vi "Project Data Initial before auto.vi"(10 "VISA resource name":refnum<visa-resource-name>="COM1", 11 "configuration file path":path=path "C:/Users/MyUser/Desktop/S2_Project.txt") -> (0 "error out":errorcluster, 1 "Step Content":string[][](table), 2 "Retry":i32, 3 "process cluster":cluster{string[], i32[]})   [LabVIEW 2019]
uses:
  <vilib>/Utility/config.llb/Read Key (String).vi
  Global/Process Global.vi
  <vilib>/Utility/config.llb/NI_LVConfig.lvlib
  Ctrl/StationCmdSelect.ctl
  FlowCtrl Class/LineScan/LineScan.lvclass
  Ctrl/MeasureDisplayTab.ctl
  LLB/Commonly VI/Main Glb.vi
  LLB/Commonly VI.lvlib
  Ctrl/Table Save.ctl
  Ctrl/Auto Inspection Station Name2.ctl
  Ctrl/Auto Inspection Data Name.ctl
  Ctrl/S2 Station IO.ctl
panel:
  out "Initial receive 2":string
  out "result string 2":string
  out "Program receive 2":string
  out "result string":string
  out "S2 receive":string
  out "Blue Scan2 receive":string
  out "T2 buffer":string
  out "T2 μA":dbl format="%#_6f"
  out "T1 buffer":string
  out "T1 μA":dbl format="%#_6f"
  in  "error in (no error)":errorcluster
  out "Blue Scan receive":string
  out "S1 receive":string
  out "Program receive":string
  out "Initial receive":string
  out "Act Step":i32
  out "retry次數":string[](array[string])
  in  "stop":bool
  out "Boolean":bool=TRUE
  in  "Numeric 3":i32
  out "format receive":string
  out "CurrentCmd":string
  out "Numeric":dbl
  out "LOG":string[][](array[string])
  in  "Enum":T1(ring)=enum."Add"
  in  "Table Control 3":string[][](table)=[["PCBA BARCODE", ""], ["硬體(Tool初始化)", ""], ["company(Tool初始化)", ""], ["耗電流 uA(電流表)", "T"], ["電池負載電壓", "T"], ["晶片ID(Tool FORMAT)", "F"], ["雷雕ID(TOOl scan、藍芽接收器)", "S"], ["Format(Tool FORMAT)", "F"], ["Programe(Tool Programe)", "P"]]
  in  "SN":string
  out "Array 3":cluster{"Table Control":string[][]}[](array[cluster])
  in  "Table Control":string[][](table)=[["PCBA BARCODE", ""], ["硬體(Tool初始化)", ""], ["company(Tool初始化)", ""], ["耗電流 uA(電流表)", "T"], ["電池負載電壓", "T"], ["晶片ID(Tool FORMAT)", "F"], ["雷雕ID(TOOl scan、藍芽接收器)", "S"], ["Format(Tool FORMAT)", "F"], ["Programe(Tool Programe)", "P"]]
  out "subarray":string[](array[string])
  out "array":string[](array[string])
  out "Process":string[](array[string])
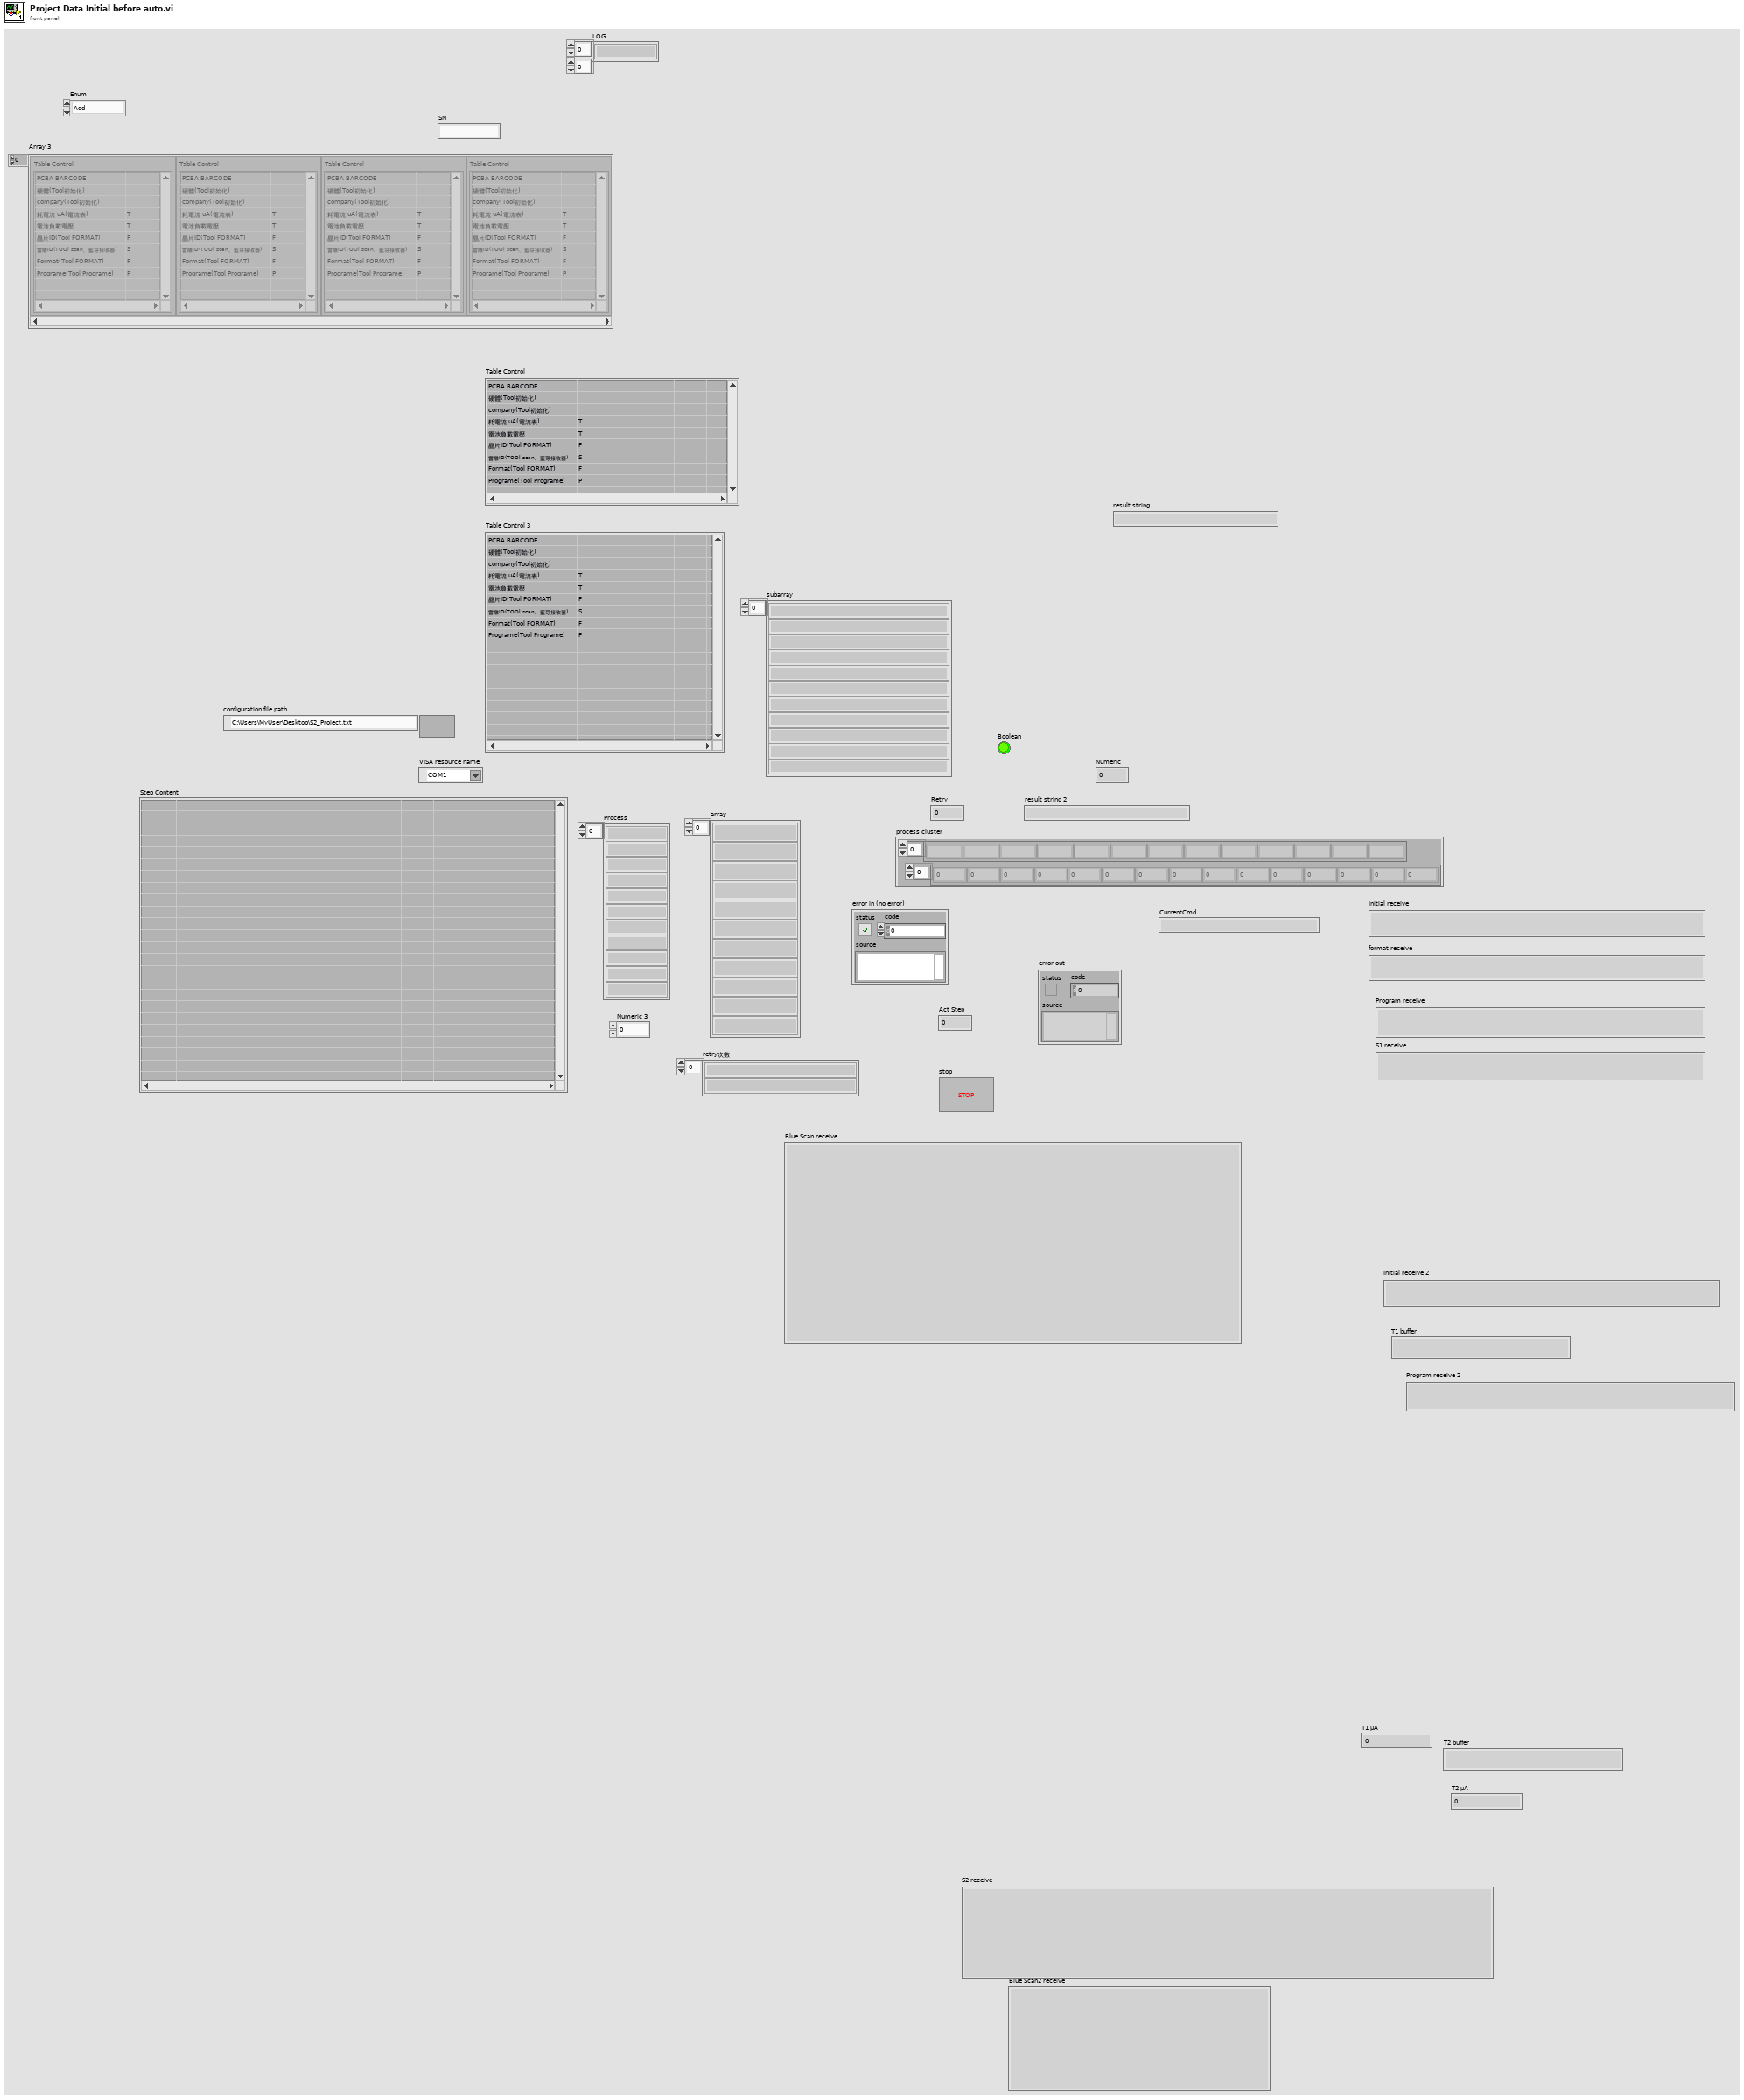
[diagram p1: front panel]
types:
  T1 = enum16{"initial", "Add", "Write", "Replace", "Delete", "REad"}
  T2 = typedef "NI_LVConfig.lvlib/Config Data RefNum.ctl" = refnum<k1>
  T3 = typedef "StationCmdSelect.ctl" = enum16{"Action", "Command", "Return", "DTime", "Retry"}
  T4 = typedef "Auto Inspection Data Name.ctl" = enum16{"LocalRun", "ItemSN(TimeCode)", "CurrentAction", "Error", "Data", "OKNG", "電壓值", "電壓值判斷", "電流值", "電流值判斷", "Laser1 Data", "Laser2 Data", "Laser OKNG", "StationNO"}
  T5 = typedef "Auto Inspection Station Name2.ctl" = enum16{"S1Barcode", "S2Measure", "S3Measure", "S4Measure", "S5Measure", "S11_LaserCheck", "S8_Vision AI"}
  T6 = typedef "Table Save.ctl" = enum16{"initial", "Add", "Write", "Replace", "Delete", "REad", "RedTable", "Load"}
  T7 = typedef "MeasureDisplayTab.ctl" = enum16{"Tray Barcode", "PCBA BARCODE", "硬體(Tool初始化)", "company(Tool初始化)", "耗電流 uA(電流表)", "電池負載電壓", "晶片ID(Tool FORMAT)", "雷雕ID(TOOl scan、藍芽接收器)", "Format(Tool FORMAT)", "Programe(Tool Programe)", "MAC(藍芽接收器)", "ID(藍芽接收器)", "KPA(藍芽接收器)", "溫度(藍芽接收器)", "SENSOR電池電壓(藍芽接收器)", "RSSI(藍芽接收器)", "SensorType_315(FSK scan)", "FSKsnVol_315(FSK scan)", "FSKscanl_315(FSK scan)", "P_315(FSK scan)", "T_315(FSK scan)", "SensorType_433(ASK scan)", "ASKsnVol_433(ASK scan)", "ASKscan_433(ASK scan)", "P_433(ASK scan)", "T_433(ASK scan)", "測高Data"}
  T8 = typedef "S2 Station IO.ctl" = enum16{"S2站PC動作中_20", "電流量測完成產品OK_21", "電流量測完成產品NG_22", "S2站Format 執行_23", "S2 Format OK_24", "S2 Format NG_25", "S2站燒入執行_26", "S2站燒入OK_27", "S2站燒入NG_28", "S2站動作完成_29", "S3 PC動作中_30", "S3 Format 此站執行_31", "S3 Format OK_32", "S3 Format NG_33", "S3 燒入程式 此站執行_34", "S3 燒入程式 OK_35", "S3 燒入程式 NG_36", "S3 備用_37", "S3 備用_38", "S3 動作完成_39", "S4 PC動作中_40", "S4 量測完成 產品正常_41", "S4 量測完成 產品NG_42", "S4 Format 此站執行_43", "S4 Format OK_44", "S4 Format NG_45", "S4 燒入 此站不執行_46", "S4 燒入程式 OK_47", "S4 燒入程式 NG_48", "S4 藍芽Scan OK_49", "S4 藍芽Scan NG_50", "S4 動作完成_51", "給PLC要量電流訊號", "給PLC要量電壓訊號"}
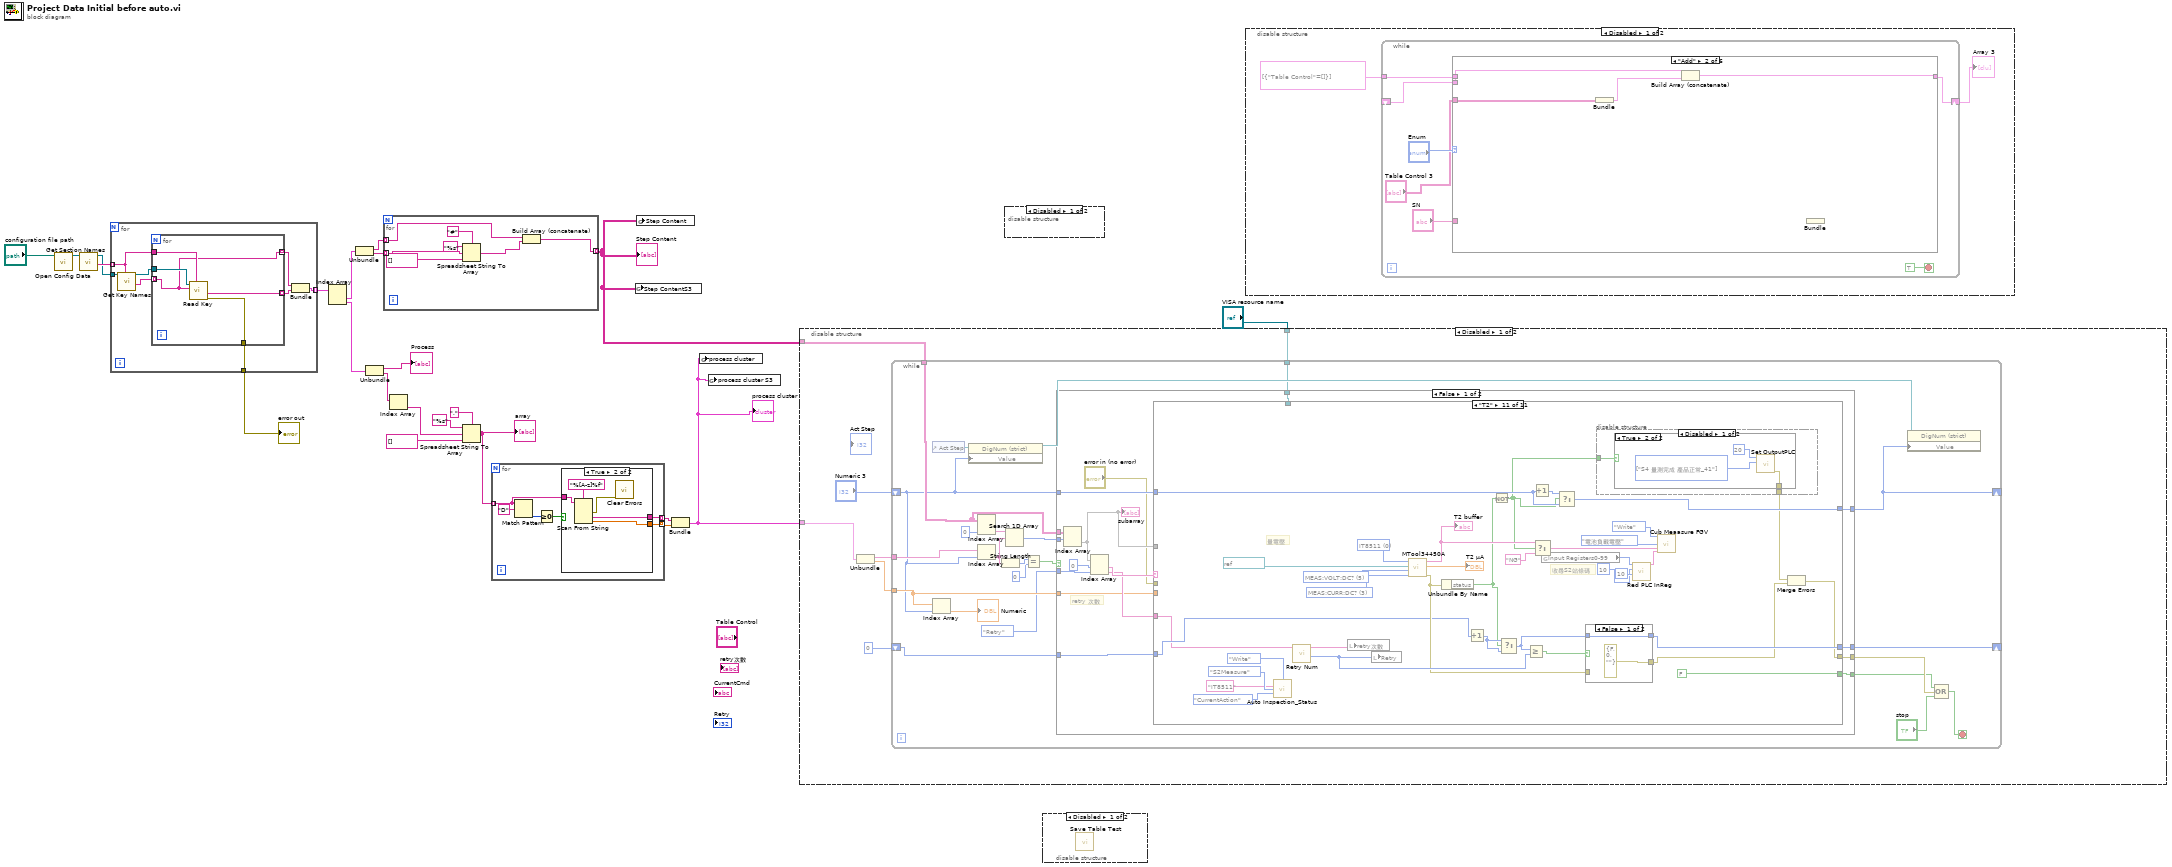
[diagram p0: block diagram]
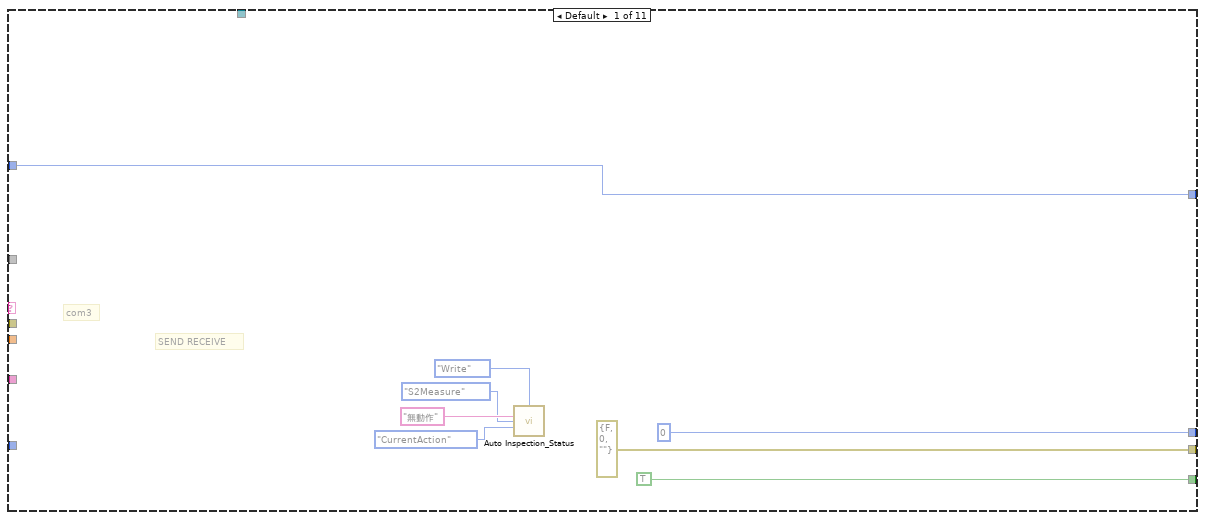
[diagram p3: hidden frame]
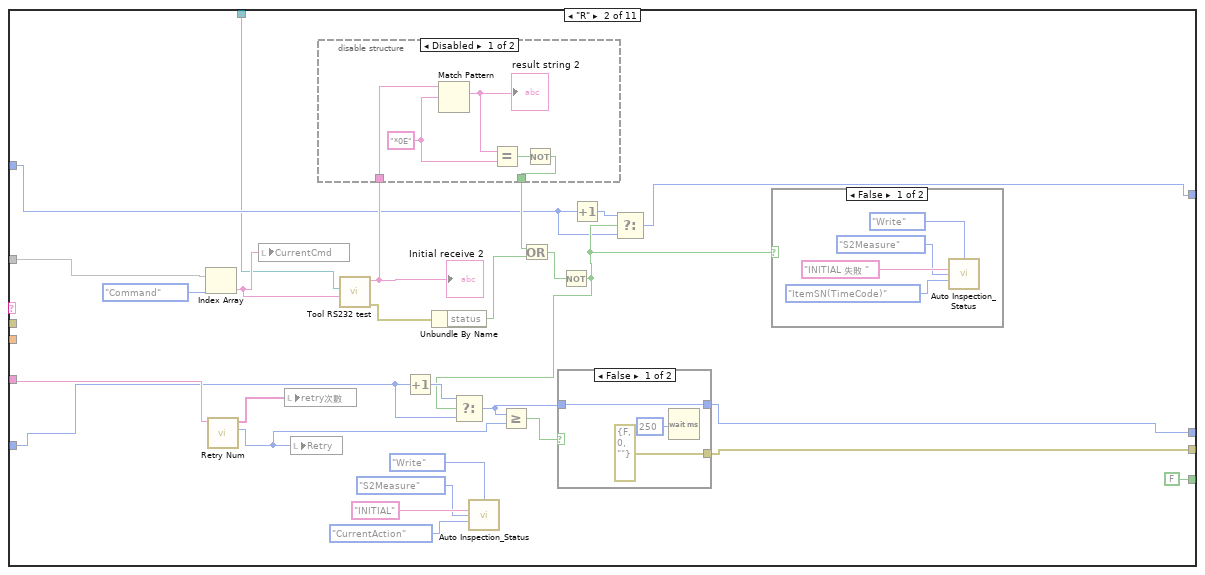
[diagram p4: hidden frame]
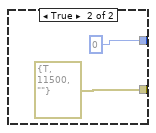
[diagram p7: hidden frame]
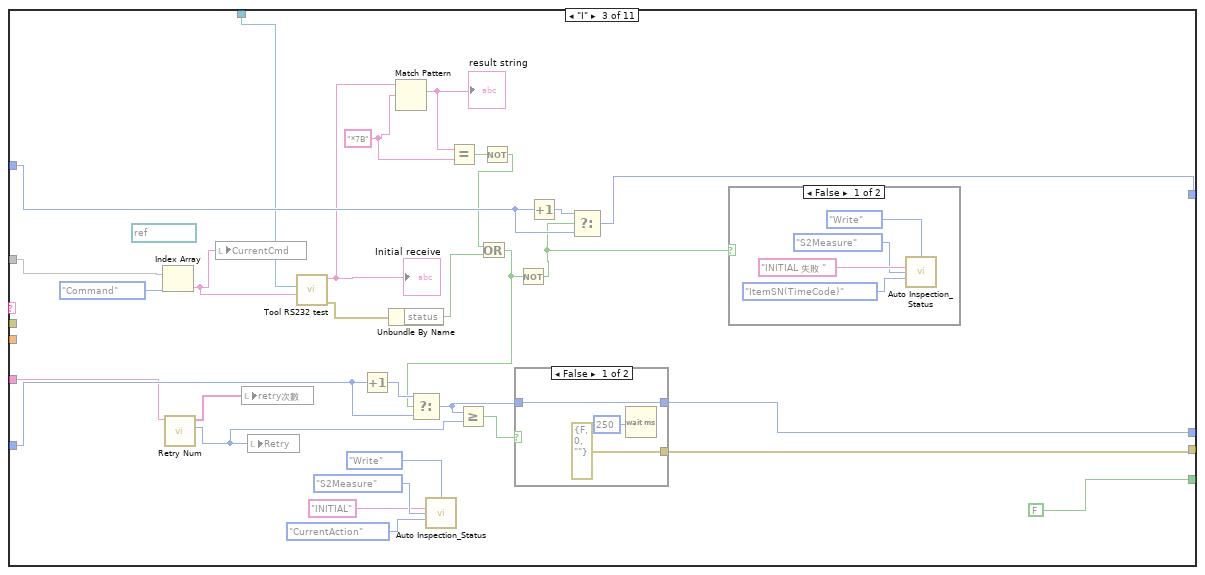
[diagram p8: hidden frame]
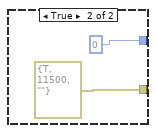
[diagram p10: hidden frame]
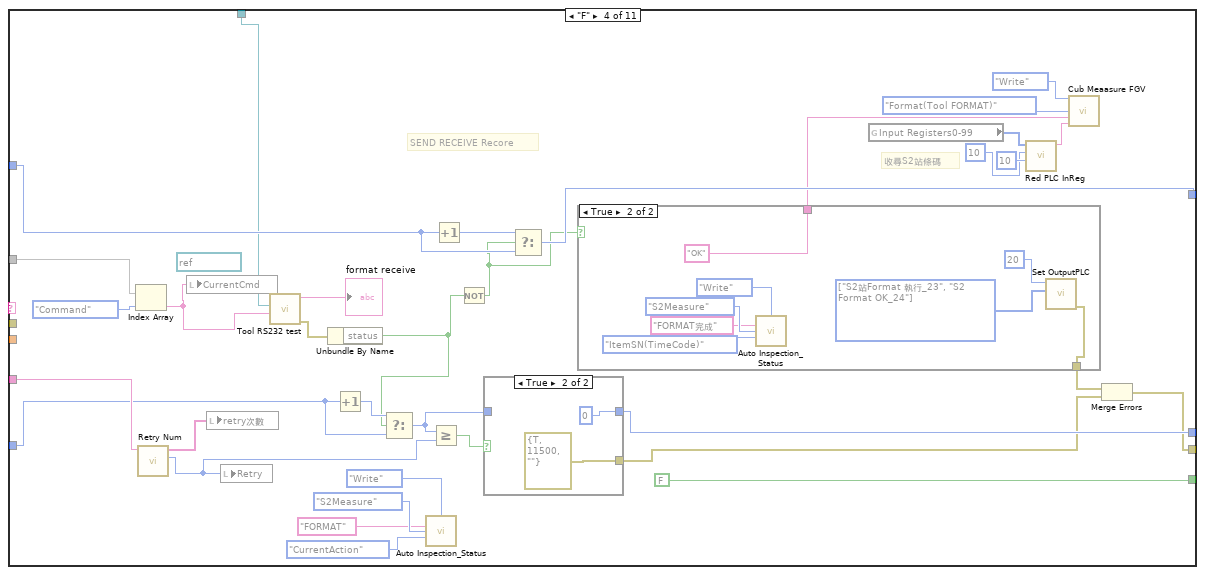
[diagram p11: hidden frame]
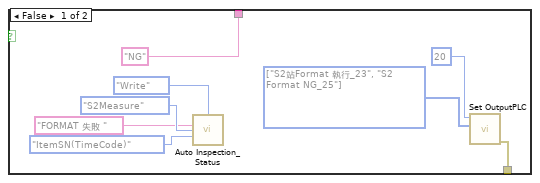
[diagram p12: hidden frame]
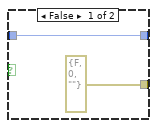
[diagram p13: hidden frame]
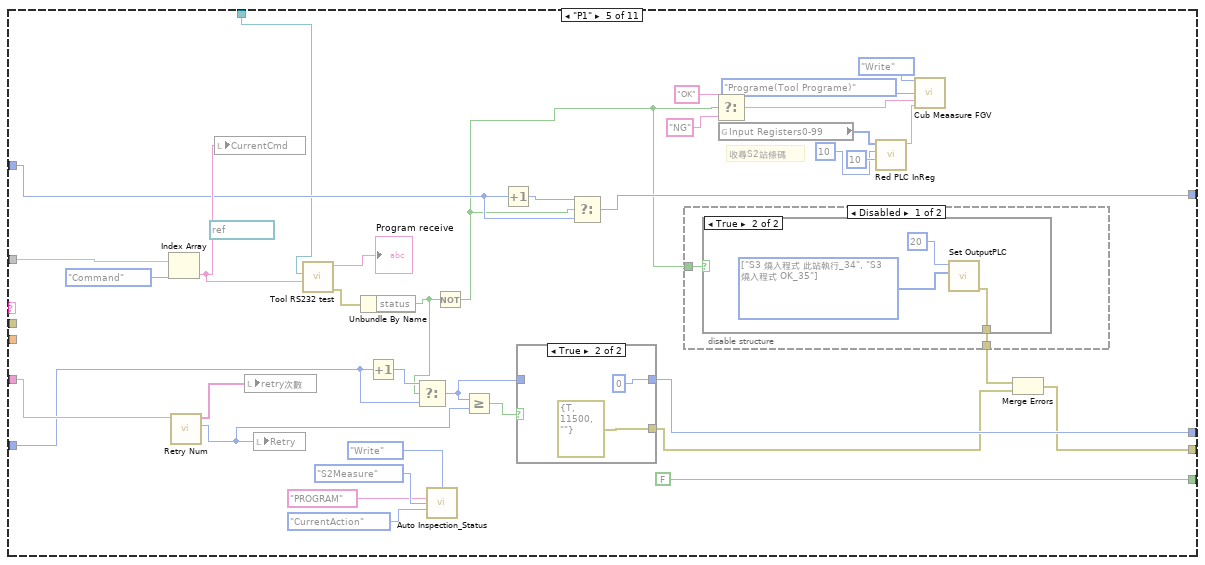
[diagram p14: hidden frame]
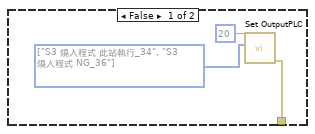
[diagram p15: hidden frame]
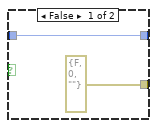
[diagram p17: hidden frame]
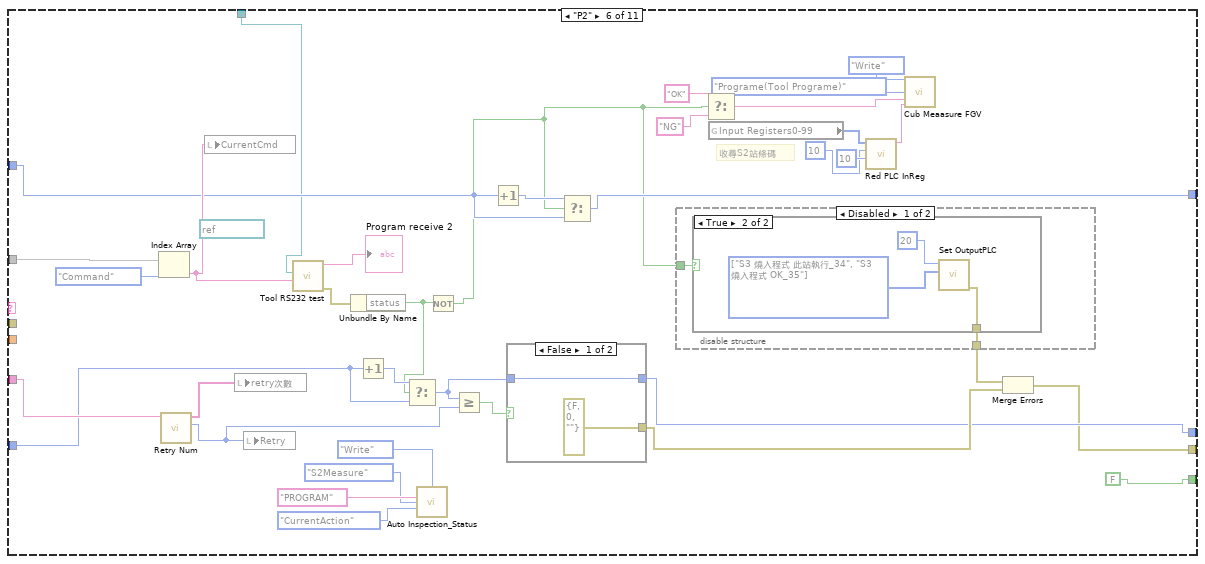
[diagram p18: hidden frame]
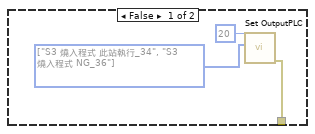
[diagram p19: hidden frame]
diagram:
  n1 = call <vilib>:"Open Config Data.vi"("configuration file path"="configuration file path") -> ("refnum"=w21:T2)  [unwired: 8 in, 2 out]
  n2 = call <vilib>:"Get Section Names.vi"("refnum"=w21) -> ("section names"=w20:string[], "refnum out"=w19:T2)  [unwired: 8 in, 1 out]
  n3 = for {
    tunnel: w19 -> [w30]
    tunnel: w20 -> [w25] mode=indexing
    tunnel: [w27] -> w17 mode=indexing
    tunnel: [w23] -> w3
    n4 = call <vilib>:"Get Key Names.vi"("section"=w25, "refnum"=w30) -> ("key names"=w29:string[], "refnum out"=w26:T2)  [unwired: 6 in, 2 out]
    n5 = for {
      tunnel: w29 -> [w32] mode=indexing
      tunnel: [w35] -> w28 mode=indexing
      tunnel: w26 -> [w34]
      tunnel: w25 -> [w33]
      tunnel: [w32] -> w24 mode=indexing
      tunnel: [w31] -> w23
      n6 = call-poly <vilib>:"Read Key.vi"("section"=w33, "key"=w32, "refnum"=w34) -> ("error out"=w31:errorcluster, "value"=w35:string)  [unwired: 5 in, 2 out]
    }
    n7 = Bundle(w24, w28) -> (w27:cluster{string[], string[]})  [unwired: 1 in]
  }
  "error out" <- w3
  n8 = Index Array(array=w17) -> (element #1=w13:cluster{string[], string[]}, element #2=w16:cluster{string[], string[]})  [unwired: 2 in]
  n9 = Unbundle(w13) -> (w14:string[], w15:string[])
  n10 = Unbundle(w16) -> (→"Process":string[], w9:string[])
  n11 = for {
    tunnel: w15 -> [w40] mode=indexing
    tunnel: [w36] -> w4 mode=indexing
    tunnel: w14 -> [w37] mode=indexing
    n12 = Spreadsheet String To Array(delimiter (Tab)="#", format string="%s", spreadsheet string=w40, array type (2D Dbl)=string[] []) -> (array=w38:string[])
    n13 = Build Array (concatenate)(w37, w38) -> (w36:string[])
  }
  "Step Content" <- w4
  n14 = Index Array(array=w9) -> (element=w8:string)  [unwired: 1 in]
  n15 = Spreadsheet String To Array(delimiter (Tab)=",", format string="%s", spreadsheet string=w8, array type (2D Dbl)=string[] []) -> (array=w7:string[])
  "array" <- w7
  n16 = for {
    tunnel: w7 -> [w43] mode=indexing
    tunnel: [w48] -> w6 mode=indexing
    tunnel: [w47] -> w5 mode=indexing
    n17 = Match Pattern(string=w43, regular expression="D") -> (offset past match=w45:i32)  [unwired: 1 in, 3 out]
    n18 = Greater Or Equal To 0?(x=w45) -> (x >= 0?=w44:bool)
    n19 = case shown="True" w44 {
      tunnel: [w50 w54] -> w48
      tunnel: [-1.0 w53] -> w47
      tunnel: w43 -> [w50 w51]
      frame False {
      }
      frame True {
        n20 = Scan From String(format string="%[A-z]%f", input string=w51) -> (error out=w52:errorcluster, output 1=w54:string, output 2=w53:dbl)  [unwired: 4 in, 2 out]
        n21 = call <vilib>:"Clear Errors.vi"("error in (no error)"=w52) -> ()  [unwired: 5 in, 2 out]
      }
    }
  }
  n22 = global write "Process Global.vi" "Step ContentS3"(w4) -> ()
  n23 = global write "Process Global.vi" "Step Content"(w4) -> ()
  n24 = Bundle(w6, w5) -> (w1:cluster{string[], dbl[]})  [unwired: 1 in]
  "process cluster" <- w1
  n25 = global write "Process Global.vi" "process cluster"(w1) -> ()
  n26 = global write "Process Global.vi" "process cluster S3"(w1) -> ()
  n27 = disable-structure shown="Disabled" {
    disable-tunnel: w4 -> [w60 _]
    disable-tunnel: w1 -> [w59 _]
    disable-tunnel: "VISA resource name" -> [w56 _]
    frame Disabled {
      n28 = Unbundle(w59) -> (w62:string[], w61:dbl[])
      n29 = while {
        tunnel: w62 -> [w85]
        tunnel: w61 -> [w84]
        tunnel: w60 -> [w83]
        shift-right: [w66] -> _
        shift-left: 0 -> [w70]
        shift-right: [w67] -> _
        shift-left: "Numeric 3" -> [w64]
        tunnel: w56 -> [w63]
        stop <- w71 stop-if-true
        n30 = control-ref of="Act Step"() -> (w69:refnum<vi>)
        n31 = Index Array(array=w84, index=w64) -> (element=→"Numeric":dbl)
        n32 = property class="DigNum (strict)"(reference=w69, "Value"=w64) -> (reference out=w68:refnum<vi>)  [unwired: 1 in, 1 out]
        n33 = Index Array(array=w83, index (col)=0 ("disabled index (col)")) -> (element=w81:string[])  [unwired: 1 in]
        n34 = Index Array(array=w85, index=w64) -> (element=w78:string)
        n35 = String Length(string=w78) -> (length=w77:i32)
        n36 = Search 1D Array(1D array=w81, element=w78) -> (index of element=w80:i32)  [unwired: 1 in]
        n37 = Equal?(x=w77, y=0) -> (x = y?=w75:bool)
        n38 = case shown="False" w75 {
          tunnel: w83 -> [w101 _]
          tunnel: w80 -> [w100 _]
          tunnel: w84 -> [w96 _]
          tunnel: w70 -> [w94 _]
          tunnel: StationCmdSelect."Retry" -> [w93 _]
          tunnel: [w92 _] -> w72
          tunnel: w64 -> [w91 _]
          tunnel: [w90 _] -> w67
          tunnel: [w89 _] -> w66
          tunnel: [w88 w564] -> w65
          tunnel: w63 -> [w86 _]
          frame False {
            # "retry 次數"
            n39 = Index Array(array=w101, index (row)=w100) -> (element=w95:string[])  [unwired: 1 in]
            "subarray" <- w95
            n40 = Index Array(array=w95, index #1=0 ("index"), index #2=w93) -> (element #1=w98:string, element #2=w97:string)
            n41 = case shown="\"T2\"" w98 {
              tunnel: w96 -> [_ _ _ _ _ _ _ _ w466 _ _]
              tunnel: w97 -> [_ w116 w168 w220 w267 w302 w367 w425 _ w488 w535]
              tunnel: w95 -> [_ w117 w170 w223 w266 w300 w364 w426 _ _ _]
              tunnel: w94 -> [_ w115 w169 w217 w264 w301 w362 w424 w463 w489 w536]
              tunnel: [errorcluster {"status"=FALSE, "code"=0, "source"=""} ("error constant") w112 w173 w193 w247 w296 w344 w403 _ w470 w519] -> w92
              tunnel: w91 -> [w109 w118 w171 w213 w263 w299 w366 w428 w461 w487 w537]
              tunnel: [w109 w111 w167 w212 w269 w298 w365 w421 w460 w486 w538] -> w90
              tunnel: [0 w114 w172 w210 w268 w297 w368 w423 _ w485 w540] -> w89
              tunnel: [TRUE FALSE FALSE FALSE FALSE FALSE FALSE FALSE FALSE FALSE FALSE] -> w88
              tunnel: "error in (no error)" -> [_ _ _ _ _ _ w341 w427 _ _ _]
              tunnel: w86 -> [_ w110 w151 w190 w244 w292 w340 w400 _ _ _]
              frame Default {
                # "SEND RECEIVE"
                # "com3"
                n42 = call "Auto Inspection_Status.vi"("Action"=enum16{"Initial", "Write", "Read"}."Write", "DataIn"="無動作", "Station"=Auto_Inspection_Station_Name2."S2Measure", "Data"=Auto_Inspection_Data_Name."CurrentAction") -> ()  [unwired: 9 in, 3 out]
              }
              frame "R" {
                n43 = Index Array(array=w117, index=StationCmdSelect."Command") -> (element=w129:string)
                n44 = call "Retry Num.vi"("String"=w116) -> ("Numeric"=w134:i32, "retry次數"=w130:string[])  [unwired: 9 in]
                n45 = local write "CurrentCmd"(w129) -> ()
                n46 = local write "retry次數"(w130) -> ()
                n47 = local write "Retry"(w134) -> ()
                n48 = call "Tool RS232 test.vi"("Cmd In"=w129, "VISA resource name"=w110) -> ("error out"=w135:errorcluster, "receive string"=w125:string)  [unwired: 8 in]
                "Initial receive 2" <- w125
                n49 = disable-structure shown="Disabled" {
                  disable-tunnel: [w140 _] -> w128
                  disable-tunnel: w125 -> [w139 _]
                  frame Disabled {
                    w137 = "*0E" ("search string")
                    n50 = Match Pattern(string=w139, regular expression=w137) -> (match substring=w138:string)  [unwired: 1 in, 3 out]
                    "result string 2" <- w138
                    n51 = Equal?(x=w138, y=w137) -> (x = y?=w141:bool)
                    n52 = Not(x=w141) -> (.not. x?=w140:bool)
                  }
                  frame Enabled {
                  }
                }
                n53 = Increment(x=w115) -> (x+1=w136:i32)
                n54 = Unbundle By Name(w135) -> ("status"=w127:bool)
                n55 = call "Auto Inspection_Status.vi"("Action"=enum16{"Initial", "Write", "Read"}."Write", "DataIn"="INITIAL", "Station"=Auto_Inspection_Station_Name2."S2Measure", "Data"=Auto_Inspection_Data_Name."CurrentAction") -> ()  [unwired: 9 in, 3 out]
                n56 = Or(x=w128, y=w127) -> (x .or. y?=w126:bool)
                n57 = Not(x=w126) -> (.not. x?=w124:bool)
                n58 = Select(t=w136, s=w124, f=w115) -> (s? t:f=w131:i32)
                n59 = Greater Or Equal?(x=w131, y=w134) -> (x >= y?=w133:bool)
                n60 = case shown="False" w133 {
                  tunnel: [errorcluster {"status"=FALSE, "code"=0, "source"=""} ("error constant") errorcluster {"status"=TRUE, "code"=11500, "source"=""} ("error constant")] -> w112
                  tunnel: w131 -> [w147 _]
                  tunnel: [w147 0] -> w114
                  frame False {
                    n61 = Wait (ms)(milliseconds to wait=250) -> ()  [unwired: 1 out]
                  }
                  frame True {
                  }
                }
                n62 = Increment(x=w118) -> (x+1=w132:i32)
                n63 = Select(t=w132, s=w124, f=w118) -> (s? t:f=w111:i32)
                n64 = case shown="False" w124 {
                  frame False {
                    n65 = call "Auto Inspection_Status.vi"("Action"=enum16{"Initial", "Write", "Read"}."Write", "DataIn"="INITIAL 失敗 ", "Station"=Auto_Inspection_Station_Name2."S2Measure", "Data"=Auto_Inspection_Data_Name."ItemSN(TimeCode)") -> ()  [unwired: 9 in, 3 out]
                  }
                  frame True {
                  }
                }
              }
              frame "I" {
                w155 = "*7B" ("search string")
                (unwired) refnum<visa-resource-name> "COM1" ("VISA resource name")
                n66 = Index Array(array=w170, index=StationCmdSelect."Command") -> (element=w165:string)
                n67 = call "Retry Num.vi"("String"=w168) -> ("Numeric"=w178:i32, "retry次數"=w166:string[])  [unwired: 9 in]
                n68 = local write "CurrentCmd"(w165) -> ()
                n69 = local write "retry次數"(w166) -> ()
                n70 = local write "Retry"(w178) -> ()
                n71 = call "Tool RS232 test.vi"("Cmd In"=w165, "VISA resource name"=w151) -> ("error out"=w179:errorcluster, "receive string"=w156:string)  [unwired: 8 in]
                "Initial receive" <- w156
                n72 = Increment(x=w169) -> (x+1=w180:i32)
                n73 = Unbundle By Name(w179) -> ("status"=w157:bool)
                n74 = Match Pattern(string=w156, regular expression=w155) -> (match substring=w154:string)  [unwired: 1 in, 3 out]
                "result string" <- w154
                n75 = call "Auto Inspection_Status.vi"("Action"=enum16{"Initial", "Write", "Read"}."Write", "DataIn"="INITIAL", "Station"=Auto_Inspection_Station_Name2."S2Measure", "Data"=Auto_Inspection_Data_Name."CurrentAction") -> ()  [unwired: 9 in, 3 out]
                n76 = Equal?(x=w154, y=w155) -> (x = y?=w159:bool)
                n77 = Not(x=w159) -> (.not. x?=w158:bool)
                n78 = Or(x=w158, y=w157) -> (x .or. y?=w152:bool)
                n79 = Select(t=w180, s=w152, f=w169) -> (s? t:f=w175:i32)
                n80 = Greater Or Equal?(x=w175, y=w178) -> (x >= y?=w177:bool)
                n81 = case shown="False" w177 {
                  tunnel: [errorcluster {"status"=FALSE, "code"=0, "source"=""} ("error constant") errorcluster {"status"=TRUE, "code"=11500, "source"=""} ("error constant")] -> w173
                  tunnel: w175 -> [w186 _]
                  tunnel: [w186 0] -> w172
                  frame False {
                    n82 = Wait (ms)(milliseconds to wait=250) -> ()  [unwired: 1 out]
                  }
                  frame True {
                  }
                }
                n83 = Not(x=w152) -> (.not. x?=w153:bool)
                n84 = Increment(x=w171) -> (x+1=w176:i32)
                n85 = Select(t=w176, s=w153, f=w171) -> (s? t:f=w167:i32)
                n86 = case shown="False" w153 {
                  frame False {
                    n87 = call "Auto Inspection_Status.vi"("Action"=enum16{"Initial", "Write", "Read"}."Write", "DataIn"="INITIAL 失敗 ", "Station"=Auto_Inspection_Station_Name2."S2Measure", "Data"=Auto_Inspection_Data_Name."ItemSN(TimeCode)") -> ()  [unwired: 9 in, 3 out]
                  }
                  frame True {
                  }
                }
              }
              frame "F" {
                (unwired) refnum<visa-resource-name> "COM1" ("VISA resource name")
                # "收尋S2站條碼"
                # "SEND RECEIVE Recore"
                n88 = Index Array(array=w223, index=StationCmdSelect."Command") -> (element=w209:string)
                n89 = call "Retry Num.vi"("String"=w220) -> ("Numeric"=w216:i32, "retry次數"=w208:string[])  [unwired: 9 in]
                n90 = local write "CurrentCmd"(w209) -> ()
                n91 = local write "retry次數"(w208) -> ()
                n92 = local write "Retry"(w216) -> ()
                n93 = call "Tool RS232 test.vi"("Cmd In"=w209, "VISA resource name"=w190) -> ("error out"=w218:errorcluster, "receive string"=→"format receive":string)  [unwired: 8 in]
                n94 = Unbundle By Name(w218) -> ("status"=w191:bool)
                n95 = Increment(x=w217) -> (x+1=w219:i32)
                n96 = Select(t=w219, s=w191, f=w217) -> (s? t:f=w211:i32)
                n97 = call "Auto Inspection_Status.vi"("Action"=enum16{"Initial", "Write", "Read"}."Write", "DataIn"="FORMAT", "Station"=Auto_Inspection_Station_Name2."S2Measure", "Data"=Auto_Inspection_Data_Name."CurrentAction") -> ()  [unwired: 9 in, 3 out]
                n98 = Greater Or Equal?(x=w211, y=w216) -> (x >= y?=w215:bool)
                n99 = Increment(x=w213) -> (x+1=w214:i32)
                n100 = Not(x=w191) -> (.not. x?=w192:bool)
                n101 = case shown="True" w215 {
                  tunnel: [errorcluster {"status"=FALSE, "code"=0, "source"=""} ("error constant") errorcluster {"status"=TRUE, "code"=11500, "source"=""} ("error constant")] -> w194
                  tunnel: w211 -> [w240 _]
                  tunnel: [w240 0] -> w210
                  frame False {
                  }
                  frame True {
                  }
                }
                n102 = Select(t=w214, s=w192, f=w213) -> (s? t:f=w212:i32)
                n103 = case shown="True" w192 {
                  tunnel: ["NG" "OK"] -> w200
                  tunnel: [w224 w232] -> w195
                  frame False {
                    w226 = T8[] [enum."S2站Format 執行_23", enum."S2 Format NG_25"] items=["S2站PC動作中_20", "電流量測完成產品OK_21", "電流量測完成產品NG_22", "S2站Format 執行_23", "S2 Format OK_24", "S2 Format NG_25", "S2站燒入執行_26", "S2站燒入OK_27", "S2站燒入NG_28", "S2站動作完成_29", "S3 PC動作中_30", "S3 Format 此站執行_31", "S3 Format OK_32", "S3 Format NG_33", "S3 燒入程式 此站執行_34", "S3 燒入程式 OK_35", "S3 燒入程式 NG_36", "S3 備用_37", "S3 備用_38", "S3 動作完成_39", "S4 PC動作中_40", "S4 量測完成 產品正常_41", "S4 量測完成 產品NG_42", "S4 Format 此站執行_43", "S4 Format OK_44", "S4 Format NG_45", "S4 燒入 此站不執行_46", "S4 燒入程式 OK_47", "S4 燒入程式 NG_48", "S4 藍芽Scan OK_49", "S4 藍芽Scan NG_50", "S4 動作完成_51", "給PLC要量電流訊號", "給PLC要量電壓訊號"]
                    n104 = call "Auto Inspection_Status.vi"("Action"=enum16{"Initial", "Write", "Read"}."Write", "DataIn"="FORMAT 失敗 ", "Station"=Auto_Inspection_Station_Name2."S2Measure", "Data"=Auto_Inspection_Data_Name."ItemSN(TimeCode)") -> ()  [unwired: 9 in, 3 out]
                    n105 = call "Set OutputPLC.vi"("Array"=w226, "Address In"=20) -> ("Error Out"=w224:errorcluster[])  [unwired: 9 in]
                  }
                  frame True {
                    w234 = T8[] [enum."S2站Format 執行_23", enum."S2 Format OK_24"] items=["S2站PC動作中_20", "電流量測完成產品OK_21", "電流量測完成產品NG_22", "S2站Format 執行_23", "S2 Format OK_24", "S2 Format NG_25", "S2站燒入執行_26", "S2站燒入OK_27", "S2站燒入NG_28", "S2站動作完成_29", "S3 PC動作中_30", "S3 Format 此站執行_31", "S3 Format OK_32", "S3 Format NG_33", "S3 燒入程式 此站執行_34", "S3 燒入程式 OK_35", "S3 燒入程式 NG_36", "S3 備用_37", "S3 備用_38", "S3 動作完成_39", "S4 PC動作中_40", "S4 量測完成 產品正常_41", "S4 量測完成 產品NG_42", "S4 Format 此站執行_43", "S4 Format OK_44", "S4 Format NG_45", "S4 燒入 此站不執行_46", "S4 燒入程式 OK_47", "S4 燒入程式 NG_48", "S4 藍芽Scan OK_49", "S4 藍芽Scan NG_50", "S4 動作完成_51", "給PLC要量電流訊號", "給PLC要量電壓訊號"]
                    n106 = call "Auto Inspection_Status.vi"("Action"=enum16{"Initial", "Write", "Read"}."Write", "DataIn"="FORMAT完成", "Station"=Auto_Inspection_Station_Name2."S2Measure", "Data"=Auto_Inspection_Data_Name."ItemSN(TimeCode)") -> ()  [unwired: 9 in, 3 out]
                    n107 = call "Set OutputPLC.vi"("Array"=w234, "Address In"=20) -> ("Error Out"=w232:errorcluster[])  [unwired: 9 in]
                  }
                }
                n108 = global read "Main Glb.vi" "Input Registers0-99"() -> (w199:u16[])
                n109 = call "Red PLC InReg.vi"("length"=10, "index"=10, "Input Registers Arr"=w199) -> ("Rad In Reg"=w196:string)  [unwired: 7 in, 1 out]
                n110 = call "Cub Meaasure FGV.vi"("Action"=Table_Save."Write" ("Enum"), 7:MeasureDisplayTab."Format(Tool FORMAT)", "DataIn"=w200, "SN"=w196) -> ()  [unwired: 5 in, 7 out]
                n111 = Merge Errors(w195, w194) -> (w193:errorcluster)
              }
              frame "P1" {
                (unwired) refnum<visa-resource-name> "COM1" ("VISA resource name")
                # "收尋S2站條碼"
                n112 = Index Array(array=w266, index=StationCmdSelect."Command") -> (element=w279:string)
                n113 = call "Retry Num.vi"("String"=w267) -> ("Numeric"=w274:i32, "retry次數"=w278:string[])  [unwired: 9 in]
                n114 = local write "CurrentCmd"(w279) -> ()
                n115 = local write "retry次數"(w278) -> ()
                n116 = local write "Retry"(w274) -> ()
                n117 = call "Tool RS232 test.vi"("Cmd In"=w279, "VISA resource name"=w244) -> ("error out"=w275:errorcluster, "receive string"=→"Program receive":string)  [unwired: 8 in]
                n118 = Unbundle By Name(w275) -> ("status"=w246:bool)
                n119 = Increment(x=w264) -> (x+1=w276:i32)
                n120 = Select(t=w276, s=w246, f=w264) -> (s? t:f=w271:i32)
                n121 = call "Auto Inspection_Status.vi"("Action"=enum16{"Initial", "Write", "Read"}."Write", "DataIn"="PROGRAM", "Station"=Auto_Inspection_Station_Name2."S2Measure", "Data"=Auto_Inspection_Data_Name."CurrentAction") -> ()  [unwired: 9 in, 3 out]
                n122 = Not(x=w246) -> (.not. x?=w245:bool)
                n123 = Greater Or Equal?(x=w271, y=w274) -> (x >= y?=w273:bool)
                n124 = Increment(x=w263) -> (x+1=w272:i32)
                n125 = case shown="True" w273 {
                  tunnel: [errorcluster {"status"=FALSE, "code"=0, "source"=""} ("error constant") errorcluster {"status"=TRUE, "code"=11500, "source"=""} ("error constant")] -> w249
                  tunnel: w271 -> [w288 _]
                  tunnel: [w288 0] -> w268
                  frame False {
                  }
                  frame True {
                  }
                }
                n126 = Select(t=w272, s=w245, f=w263) -> (s? t:f=w269:i32)
                n127 = disable-structure shown="Disabled" {
                  disable-tunnel: w245 -> [w281 _]
                  disable-tunnel: [w280 _] -> w248
                  frame Disabled {
                    n128 = case shown="True" w281 {
                      tunnel: [w282 w285] -> w280
                      frame False {
                        w284 = T8[] [enum."S3 燒入程式 此站執行_34", enum."S3 燒入程式 NG_36"] items=["S2站PC動作中_20", "電流量測完成產品OK_21", "電流量測完成產品NG_22", "S2站Format 執行_23", "S2 Format OK_24", "S2 Format NG_25", "S2站燒入執行_26", "S2站燒入OK_27", "S2站燒入NG_28", "S2站動作完成_29", "S3 PC動作中_30", "S3 Format 此站執行_31", "S3 Format OK_32", "S3 Format NG_33", "S3 燒入程式 此站執行_34", "S3 燒入程式 OK_35", "S3 燒入程式 NG_36", "S3 備用_37", "S3 備用_38", "S3 動作完成_39", "S4 PC動作中_40", "S4 量測完成 產品正常_41", "S4 量測完成 產品NG_42", "S4 Format 此站執行_43", "S4 Format OK_44", "S4 Format NG_45", "S4 燒入 此站不執行_46", "S4 燒入程式 OK_47", "S4 燒入程式 NG_48", "S4 藍芽Scan OK_49", "S4 藍芽Scan NG_50", "S4 動作完成_51", "給PLC要量電流訊號", "給PLC要量電壓訊號"]
                        n129 = call "Set OutputPLC.vi"("Array"=w284, "Address In"=20) -> ("Error Out"=w282:errorcluster[])  [unwired: 9 in]
                      }
                      frame True {
                        w286 = T8[] [enum."S3 燒入程式 此站執行_34", enum."S3 燒入程式 OK_35"] items=["S2站PC動作中_20", "電流量測完成產品OK_21", "電流量測完成產品NG_22", "S2站Format 執行_23", "S2 Format OK_24", "S2 Format NG_25", "S2站燒入執行_26", "S2站燒入OK_27", "S2站燒入NG_28", "S2站動作完成_29", "S3 PC動作中_30", "S3 Format 此站執行_31", "S3 Format OK_32", "S3 Format NG_33", "S3 燒入程式 此站執行_34", "S3 燒入程式 OK_35", "S3 燒入程式 NG_36", "S3 備用_37", "S3 備用_38", "S3 動作完成_39", "S4 PC動作中_40", "S4 量測完成 產品正常_41", "S4 量測完成 產品NG_42", "S4 Format 此站執行_43", "S4 Format OK_44", "S4 Format NG_45", "S4 燒入 此站不執行_46", "S4 燒入程式 OK_47", "S4 燒入程式 NG_48", "S4 藍芽Scan OK_49", "S4 藍芽Scan NG_50", "S4 動作完成_51", "給PLC要量電流訊號", "給PLC要量電壓訊號"]
                        n130 = call "Set OutputPLC.vi"("Array"=w286, "Address In"=20) -> ("Error Out"=w285:errorcluster[])  [unwired: 9 in]
                      }
                    }
                  }
                  frame Enabled {
                  }
                }
                n131 = Select(t="OK" ("DataIn"), s=w245, f="NG" ("DataIn")) -> (s? t:f=w250:string)
                n132 = global read "Main Glb.vi" "Input Registers0-99"() -> (w258:u16[])
                n133 = call "Red PLC InReg.vi"("length"=10, "index"=10, "Input Registers Arr"=w258) -> ("Rad In Reg"=w257:string)  [unwired: 7 in, 1 out]
                n134 = call "Cub Meaasure FGV.vi"("Action"=Table_Save."Write" ("Enum"), 7:MeasureDisplayTab."Programe(Tool Programe)", "DataIn"=w250, "SN"=w257) -> ()  [unwired: 5 in, 7 out]
                n135 = Merge Errors(w248, w249) -> (w247:errorcluster)
              }
              frame "P2" {
                (unwired) refnum<visa-resource-name> "COM1" ("VISA resource name")
                # "收尋S2站條碼"
                n136 = Index Array(array=w300, index=StationCmdSelect."Command") -> (element=w327:string)
                n137 = call "Retry Num.vi"("String"=w302) -> ("Numeric"=w322:i32, "retry次數"=w326:string[])  [unwired: 9 in]
                n138 = local write "CurrentCmd"(w327) -> ()
                n139 = local write "retry次數"(w326) -> ()
                n140 = local write "Retry"(w322) -> ()
                n141 = call "Tool RS232 test.vi"("Cmd In"=w327, "VISA resource name"=w292) -> ("error out"=w323:errorcluster, "receive string"=→"Program receive 2":string)  [unwired: 8 in]
                n142 = Unbundle By Name(w323) -> ("status"=w293:bool)
                n143 = Increment(x=w301) -> (x+1=w324:i32)
                n144 = Select(t=w324, s=w293, f=w301) -> (s? t:f=w319:i32)
                n145 = call "Auto Inspection_Status.vi"("Action"=enum16{"Initial", "Write", "Read"}."Write", "DataIn"="PROGRAM", "Station"=Auto_Inspection_Station_Name2."S2Measure", "Data"=Auto_Inspection_Data_Name."CurrentAction") -> ()  [unwired: 9 in, 3 out]
                n146 = Not(x=w293) -> (.not. x?=w294:bool)
                n147 = Greater Or Equal?(x=w319, y=w322) -> (x >= y?=w321:bool)
                n148 = Increment(x=w299) -> (x+1=w320:i32)
                n149 = case shown="False" w321 {
                  tunnel: [errorcluster {"status"=FALSE, "code"=0, "source"=""} ("error constant") errorcluster {"status"=TRUE, "code"=11500, "source"=""} ("error constant")] -> w315
                  tunnel: w319 -> [w336 _]
                  tunnel: [w336 0] -> w297
                  frame False {
                  }
                  frame True {
                  }
                }
                n150 = Select(t=w320, s=w294, f=w299) -> (s? t:f=w298:i32)
                n151 = disable-structure shown="Disabled" {
                  disable-tunnel: [w329 _] -> w314
                  disable-tunnel: w294 -> [w328 _]
                  frame Disabled {
                    n152 = case shown="True" w328 {
                      tunnel: [w330 w333] -> w329
                      frame False {
                        w332 = T8[] [enum."S3 燒入程式 此站執行_34", enum."S3 燒入程式 NG_36"] items=["S2站PC動作中_20", "電流量測完成產品OK_21", "電流量測完成產品NG_22", "S2站Format 執行_23", "S2 Format OK_24", "S2 Format NG_25", "S2站燒入執行_26", "S2站燒入OK_27", "S2站燒入NG_28", "S2站動作完成_29", "S3 PC動作中_30", "S3 Format 此站執行_31", "S3 Format OK_32", "S3 Format NG_33", "S3 燒入程式 此站執行_34", "S3 燒入程式 OK_35", "S3 燒入程式 NG_36", "S3 備用_37", "S3 備用_38", "S3 動作完成_39", "S4 PC動作中_40", "S4 量測完成 產品正常_41", "S4 量測完成 產品NG_42", "S4 Format 此站執行_43", "S4 Format OK_44", "S4 Format NG_45", "S4 燒入 此站不執行_46", "S4 燒入程式 OK_47", "S4 燒入程式 NG_48", "S4 藍芽Scan OK_49", "S4 藍芽Scan NG_50", "S4 動作完成_51", "給PLC要量電流訊號", "給PLC要量電壓訊號"]
                        n153 = call "Set OutputPLC.vi"("Array"=w332, "Address In"=20) -> ("Error Out"=w330:errorcluster[])  [unwired: 9 in]
                      }
                      frame True {
                        w334 = T8[] [enum."S3 燒入程式 此站執行_34", enum."S3 燒入程式 OK_35"] items=["S2站PC動作中_20", "電流量測完成產品OK_21", "電流量測完成產品NG_22", "S2站Format 執行_23", "S2 Format OK_24", "S2 Format NG_25", "S2站燒入執行_26", "S2站燒入OK_27", "S2站燒入NG_28", "S2站動作完成_29", "S3 PC動作中_30", "S3 Format 此站執行_31", "S3 Format OK_32", "S3 Format NG_33", "S3 燒入程式 此站執行_34", "S3 燒入程式 OK_35", "S3 燒入程式 NG_36", "S3 備用_37", "S3 備用_38", "S3 動作完成_39", "S4 PC動作中_40", "S4 量測完成 產品正常_41", "S4 量測完成 產品NG_42", "S4 Format 此站執行_43", "S4 Format OK_44", "S4 Format NG_45", "S4 燒入 此站不執行_46", "S4 燒入程式 OK_47", "S4 燒入程式 NG_48", "S4 藍芽Scan OK_49", "S4 藍芽Scan NG_50", "S4 動作完成_51", "給PLC要量電流訊號", "給PLC要量電壓訊號"]
                        n154 = call "Set OutputPLC.vi"("Array"=w334, "Address In"=20) -> ("Error Out"=w333:errorcluster[])  [unwired: 9 in]
                      }
                    }
                  }
                  frame Enabled {
                  }
                }
                n155 = Select(t="OK" ("DataIn"), s=w294, f="NG" ("DataIn")) -> (s? t:f=w316:string)
                n156 = global read "Main Glb.vi" "Input Registers0-99"() -> (w318:u16[])
                n157 = call "Red PLC InReg.vi"("length"=10, "index"=10, "Input Registers Arr"=w318) -> ("Rad In Reg"=w317:string)  [unwired: 7 in, 1 out]
                n158 = call "Cub Meaasure FGV.vi"("Action"=Table_Save."Write" ("Enum"), 7:MeasureDisplayTab."Programe(Tool Programe)", "DataIn"=w316, "SN"=w317) -> ()  [unwired: 5 in, 7 out]
                n159 = Merge Errors(w314, w315) -> (w296:errorcluster)
              }
              frame "S1" {
                # "收尋S2站條碼"
                # "SEND RECEIVE Recore"
                n160 = disable-structure shown="Enabled" {
                  disable-tunnel: [w382 _] -> w361
                  disable-tunnel: w341 -> [w381 _]
                  frame Enabled {
                    n161 = call "wait.vi"("error in"=w381, "wait(ms)"=100) -> ("error out"=w380:errorcluster)  [unwired: 9 in]
                    n162 = call "ToolScanTest.vi"("error in (no error)"=w380, "VISA resource name"=refnum<visa-resource-name> "COM10") -> ("error out"=w386:errorcluster, "read string 6"=w383:string)  [unwired: 4 in, 4 out]
                    "Blue Scan receive" <- w383
                    n163 = call <vilib>:"Clear Errors.vi"("error in (no error)"=w386) -> ()  [unwired: 5 in, 2 out]
                    n164 = String Length(string=w383) -> (length=w385:i32)
                    n165 = Not Equal To 0?(x=w385) -> (x != 0?=w384:bool)
                    n166 = Not(x=w384) -> (.not. x?=w382:bool)
                  }
                  frame Disabled {
                  }
                }
                n167 = Index Array(array=w364, index=StationCmdSelect."Command") -> (element=w377:string)
                n168 = call "Retry Num.vi"("String"=w367) -> ("Numeric"=w372:i32, "retry次數"=w376:string[])  [unwired: 9 in]
                n169 = local write "CurrentCmd"(w377) -> ()
                n170 = local write "retry次數"(w376) -> ()
                n171 = local write "Retry"(w372) -> ()
                n172 = call "Tool RS232 test.vi"("error in (no error)"=w341, "Cmd In"=w377, "VISA resource name"=w340) -> ("error out"=w373:errorcluster, "receive string"=→"S1 receive":string)  [unwired: 7 in]
                n173 = Unbundle By Name(w373) -> ("status"=w360:bool)
                n174 = Increment(x=w362) -> (x+1=w374:i32)
                n175 = call "Auto Inspection_Status.vi"("Action"=enum16{"Initial", "Write", "Read"}."Write", "DataIn"="SCAN1", "Station"=Auto_Inspection_Station_Name2."S2Measure", "Data"=Auto_Inspection_Data_Name."CurrentAction") -> ()  [unwired: 9 in, 3 out]
                n176 = Or(x=w361, y=w360) -> (x .or. y?=w342:bool)
                n177 = Select(t=w374, s=w342, f=w362) -> (s? t:f=w369:i32)
                n178 = Greater Or Equal?(x=w369, y=w372) -> (x >= y?=w371:bool)
                n179 = Not(x=w342) -> (.not. x?=w343:bool)
                n180 = case shown="False" w371 {
                  tunnel: [errorcluster {"status"=FALSE, "code"=0, "source"=""} ("error constant") errorcluster {"status"=TRUE, "code"=11500, "source"=""} ("error constant")] -> w345
                  tunnel: w369 -> [w396 _]
                  tunnel: [w396 0] -> w368
                  frame False {
                  }
                  frame True {
                  }
                }
                n181 = Increment(x=w366) -> (x+1=w370:i32)
                n182 = Select(t=w370, s=w343, f=w366) -> (s? t:f=w365:i32)
                n183 = disable-structure shown="Disabled" {
                  disable-tunnel: [w389 _] -> w346
                  disable-tunnel: w343 -> [w388 _]
                  frame Disabled {
                    n184 = case shown="False" w388 {
                      tunnel: [w390 w394] -> w389
                      frame False {
                        w392 = T8[] [enum."S4 量測完成 產品NG_42"] items=["S2站PC動作中_20", "電流量測完成產品OK_21", "電流量測完成產品NG_22", "S2站Format 執行_23", "S2 Format OK_24", "S2 Format NG_25", "S2站燒入執行_26", "S2站燒入OK_27", "S2站燒入NG_28", "S2站動作完成_29", "S3 PC動作中_30", "S3 Format 此站執行_31", "S3 Format OK_32", "S3 Format NG_33", "S3 燒入程式 此站執行_34", "S3 燒入程式 OK_35", "S3 燒入程式 NG_36", "S3 備用_37", "S3 備用_38", "S3 動作完成_39", "S4 PC動作中_40", "S4 量測完成 產品正常_41", "S4 量測完成 產品NG_42", "S4 Format 此站執行_43", "S4 Format OK_44", "S4 Format NG_45", "S4 燒入 此站不執行_46", "S4 燒入程式 OK_47", "S4 燒入程式 NG_48", "S4 藍芽Scan OK_49", "S4 藍芽Scan NG_50", "S4 動作完成_51", "給PLC要量電流訊號", "給PLC要量電壓訊號"]
                        n185 = call "Set OutputPLC.vi"("Array"=w392, "Address In"=20) -> ("Error Out"=w390:errorcluster[])  [unwired: 9 in]
                      }
                      frame True {
                        w393 = T8[] [enum."S4 量測完成 產品正常_41"] items=["S2站PC動作中_20", "電流量測完成產品OK_21", "電流量測完成產品NG_22", "S2站Format 執行_23", "S2 Format OK_24", "S2 Format NG_25", "S2站燒入執行_26", "S2站燒入OK_27", "S2站燒入NG_28", "S2站動作完成_29", "S3 PC動作中_30", "S3 Format 此站執行_31", "S3 Format OK_32", "S3 Format NG_33", "S3 燒入程式 此站執行_34", "S3 燒入程式 OK_35", "S3 燒入程式 NG_36", "S3 備用_37", "S3 備用_38", "S3 動作完成_39", "S4 PC動作中_40", "S4 量測完成 產品正常_41", "S4 量測完成 產品NG_42", "S4 Format 此站執行_43", "S4 Format OK_44", "S4 Format NG_45", "S4 燒入 此站不執行_46", "S4 燒入程式 OK_47", "S4 燒入程式 NG_48", "S4 藍芽Scan OK_49", "S4 藍芽Scan NG_50", "S4 動作完成_51", "給PLC要量電流訊號", "給PLC要量電壓訊號"]
                        n186 = call "Set OutputPLC.vi"("Array"=w393, "Address In"=20) -> ("Error Out"=w394:errorcluster[])  [unwired: 9 in]
                      }
                    }
                  }
                  frame Enabled {
                  }
                }
                n187 = global read "Main Glb.vi" "Input Registers0-99"() -> (w355:u16[])
                n188 = Select(t="OK" ("DataIn"), s=w343, f="NG" ("DataIn")) -> (s? t:f=w347:string)
                n189 = call "Red PLC InReg.vi"("length"=10, "index"=10, "Input Registers Arr"=w355) -> ("Rad In Reg"=w354:string)  [unwired: 7 in, 1 out]
                n190 = call "Cub Meaasure FGV.vi"("Action"=Table_Save."Write" ("Enum"), 7:MeasureDisplayTab."FSKscanl_315(FSK scan)", "DataIn"=w347, "SN"=w354) -> ()  [unwired: 5 in, 7 out]
                n191 = Merge Errors(w346, w345) -> (w344:errorcluster)
              }
              frame "S2" {
                (unwired) refnum<visa-resource-name> "COM1" ("VISA resource name")
                # "收尋S2站條碼"
                n192 = call "Retry Num.vi"("String"=w425) -> ("Numeric"=w439:i32, "retry次數"=w436:string[])  [unwired: 9 in]
                n193 = Index Array(array=w426, index=StationCmdSelect."Command") -> (element=w419:string)
                n194 = call "ToolScanTest.vi"("error in (no error)"=w427, "VISA resource name"=refnum<visa-resource-name> "COM10") -> ("error out"=w435:errorcluster, "read string 6"=w420:string)  [unwired: 4 in, 4 out]
                "Blue Scan2 receive" <- w420
                n195 = local write "retry次數"(w436) -> ()
                n196 = call "Tool RS232 test.vi"("error in (no error)"=w427, "Cmd In"=w419, "VISA resource name"=w400) -> ("error out"=w442:errorcluster, "receive string"=→"S2 receive":string)  [unwired: 7 in]
                n197 = call <vilib>:"Clear Errors.vi"("error in (no error)"=w435) -> ()  [unwired: 5 in, 2 out]
                n198 = local write "CurrentCmd"(w419) -> ()
                n199 = local write "Retry"(w439) -> ()
                n200 = Unbundle By Name(w442) -> ("status"=w431:bool)
                n201 = String Length(string=w420) -> (length=w434:i32)
                n202 = Not Equal To 0?(x=w434) -> (x != 0?=w433:bool)
                n203 = Not(x=w433) -> (.not. x?=w432:bool)
                n204 = Or(x=w432, y=w431) -> (x .or. y?=w401:bool)
                n205 = Not(x=w401) -> (.not. x?=w402:bool)
                n206 = call "Auto Inspection_Status.vi"("Action"=enum16{"Initial", "Write", "Read"}."Write", "DataIn"="SCAN2", "Station"=Auto_Inspection_Station_Name2."S2Measure", "Data"=Auto_Inspection_Data_Name."CurrentAction") -> ()  [unwired: 9 in, 3 out]
                n207 = Increment(x=w424) -> (x+1=w440:i32)
                n208 = Select(t=w440, s=w401, f=w424) -> (s? t:f=w437:i32)
                n209 = Increment(x=w428) -> (x+1=w441:i32)
                n210 = Greater Or Equal?(x=w437, y=w439) -> (x >= y?=w438:bool)
                n211 = Select(t=w441, s=w402, f=w428) -> (s? t:f=w421:i32)
                n212 = case shown="True" w438 {
                  tunnel: [errorcluster {"status"=FALSE, "code"=0, "source"=""} ("error constant") errorcluster {"status"=TRUE, "code"=11505, "source"=""} ("error constant")] -> w404
                  tunnel: w437 -> [w452 _]
                  tunnel: [w452 0] -> w423
                  frame False {
                  }
                  frame True {
                  }
                }
                n213 = disable-structure shown="Disabled" {
                  disable-tunnel: [w445 _] -> w405
                  disable-tunnel: w402 -> [w444 _]
                  frame Disabled {
                    n214 = case shown="False" w444 {
                      tunnel: [w446 w450] -> w445
                      frame False {
                        w448 = T8[] [enum."S4 量測完成 產品NG_42"] items=["S2站PC動作中_20", "電流量測完成產品OK_21", "電流量測完成產品NG_22", "S2站Format 執行_23", "S2 Format OK_24", "S2 Format NG_25", "S2站燒入執行_26", "S2站燒入OK_27", "S2站燒入NG_28", "S2站動作完成_29", "S3 PC動作中_30", "S3 Format 此站執行_31", "S3 Format OK_32", "S3 Format NG_33", "S3 燒入程式 此站執行_34", "S3 燒入程式 OK_35", "S3 燒入程式 NG_36", "S3 備用_37", "S3 備用_38", "S3 動作完成_39", "S4 PC動作中_40", "S4 量測完成 產品正常_41", "S4 量測完成 產品NG_42", "S4 Format 此站執行_43", "S4 Format OK_44", "S4 Format NG_45", "S4 燒入 此站不執行_46", "S4 燒入程式 OK_47", "S4 燒入程式 NG_48", "S4 藍芽Scan OK_49", "S4 藍芽Scan NG_50", "S4 動作完成_51", "給PLC要量電流訊號", "給PLC要量電壓訊號"]
                        n215 = call "Set OutputPLC.vi"("Array"=w448, "Address In"=20) -> ("Error Out"=w446:errorcluster[])  [unwired: 9 in]
                      }
                      frame True {
                        w449 = T8[] [enum."S4 量測完成 產品正常_41"] items=["S2站PC動作中_20", "電流量測完成產品OK_21", "電流量測完成產品NG_22", "S2站Format 執行_23", "S2 Format OK_24", "S2 Format NG_25", "S2站燒入執行_26", "S2站燒入OK_27", "S2站燒入NG_28", "S2站動作完成_29", "S3 PC動作中_30", "S3 Format 此站執行_31", "S3 Format OK_32", "S3 Format NG_33", "S3 燒入程式 此站執行_34", "S3 燒入程式 OK_35", "S3 燒入程式 NG_36", "S3 備用_37", "S3 備用_38", "S3 動作完成_39", "S4 PC動作中_40", "S4 量測完成 產品正常_41", "S4 量測完成 產品NG_42", "S4 Format 此站執行_43", "S4 Format OK_44", "S4 Format NG_45", "S4 燒入 此站不執行_46", "S4 燒入程式 OK_47", "S4 燒入程式 NG_48", "S4 藍芽Scan OK_49", "S4 藍芽Scan NG_50", "S4 動作完成_51", "給PLC要量電流訊號", "給PLC要量電壓訊號"]
                        n216 = call "Set OutputPLC.vi"("Array"=w449, "Address In"=20) -> ("Error Out"=w450:errorcluster[])  [unwired: 9 in]
                      }
                    }
                  }
                  frame Enabled {
                  }
                }
                n217 = Select(t="OK" ("DataIn"), s=w402, f="NG" ("DataIn")) -> (s? t:f=w406:string)
                n218 = global read "Main Glb.vi" "Input Registers0-99"() -> (w414:u16[])
                n219 = call "Red PLC InReg.vi"("length"=10, "index"=10, "Input Registers Arr"=w414) -> ("Rad In Reg"=w413:string)  [unwired: 7 in, 1 out]
                n220 = call "Cub Meaasure FGV.vi"("Action"=Table_Save."Write" ("Enum"), 7:MeasureDisplayTab."ASKscan_433(ASK scan)", "DataIn"=w406, "SN"=w413) -> ()  [unwired: 5 in, 7 out]
                n221 = Merge Errors(w405, w404) -> (w403:errorcluster)
              }
              frame "D" {
                n222 = Index Array(array=w466, index=w463) -> (element=w465:dbl)
                n223 = Multiply(x=1000, y=w465) -> (x*y=w464:dbl)
                n224 = Wait (ms)(milliseconds to wait=w464) -> ()  [unwired: 1 out]
                n225 = call "Auto Inspection_Status.vi"("Action"=enum16{"Initial", "Write", "Read"}."Write", "DataIn"="Delay Time", "Station"=Auto_Inspection_Station_Name2."S2Measure", "Data"=Auto_Inspection_Data_Name."CurrentAction") -> ()  [unwired: 9 in, 3 out]
                n226 = Increment(x=w461) -> (x+1=w460:i32)
              }
              frame "T1" {
                (unwired) 10 ("index")
                w493 = u16 3 items=["SYSTem:VERSion?", "SYSTem:ERRor?", "*IDN?", "MEAS:CURR:DC?", "MEAS:VOLT?", "SYSTem:ERRor?"] ("Ringfor34450A")
                w492 = u16 5 items=["SYSTem:VERSion?", "SYSTem:ERRor?", "*IDN?", "MEAS:CURR:DC?", "MEAS:VOLT?", "MEAS:VOLT:DC?"] ("RingforIT8511")
                w490 = u16 1 items=["IT8511", "34450A", "WRBuff"] ("ChangeStatus")
                # "收尋S2站條碼"
                # "量電流"
                n227 = call "Retry Num.vi"("String"=w488) -> ("Numeric"=w498:i32, "retry次數"=w497:string[])  [unwired: 9 in]
                n228 = local write "retry次數"(w497) -> ()
                n229 = call "Auto Inspection_Status.vi"("Action"=enum16{"Initial", "Write", "Read"}."Write", "DataIn"="儀器34450A", "Station"=Auto_Inspection_Station_Name2."S2Measure", "Data"=Auto_Inspection_Data_Name."CurrentAction") -> ()  [unwired: 9 in, 3 out]
                n230 = local write "Retry"(w498) -> ()
                n231 = call "MTool34450A.vi"("Ringfor34450A"=w493, "RingforIT8511"=w492, "VISA resource name"=refnum<visa-resource-name> "USB0::0x2A8D::0xB318::MY59430005::INSTR", "ChangeStatus"=w490) -> ("error out"=w494:errorcluster, 1:"μA"=w473:string, 2:"μA"=→"T1 μA":dbl, "read buffer"=→"T1 buffer":string)  [unwired: 4 in]
                n232 = Unbundle By Name(w494) -> ("status"=w468:bool)
                n233 = Increment(x=w489) -> (x+1=w499:i32)
                n234 = Not(x=w468) -> (.not. x?=w469:bool)
                n235 = Select(t=w499, s=w468, f=w489) -> (s? t:f=w496:i32)
                n236 = Greater Or Equal?(x=w496, y=w498) -> (x >= y?=w495:bool)
                n237 = Increment(x=w487) -> (x+1=w500:i32)
                n238 = Select(t=w500, s=w469, f=w487) -> (s? t:f=w486:i32)
                n239 = case shown="False" w495 {
                  tunnel: [errorcluster {"status"=FALSE, "code"=0, "source"=""} ("error constant") w514] -> w471
                  tunnel: w496 -> [w512 _]
                  tunnel: [w512 0] -> w485
                  tunnel: w494 -> [_ w514]
                  frame False {
                  }
                  frame True {
                  }
                }
                n240 = Select(t=w473, s=w469, f="NG" ("DataIn")) -> (s? t:f=w474:string)
                n241 = global read "Main Glb.vi" "Input Registers0-99"() -> (w480:u16[])
                n242 = disable-structure shown="Disabled" {
                  disable-tunnel: [w505 _] -> w472
                  disable-tunnel: w469 -> [w504 _]
                  frame Disabled {
                    n243 = case shown="True" w504 {
                      tunnel: [w506 w509] -> w505
                      frame False {
                        w508 = T8[] [enum."電流量測完成產品NG_22"] items=["S2站PC動作中_20", "電流量測完成產品OK_21", "電流量測完成產品NG_22", "S2站Format 執行_23", "S2 Format OK_24", "S2 Format NG_25", "S2站燒入執行_26", "S2站燒入OK_27", "S2站燒入NG_28", "S2站動作完成_29", "S3 PC動作中_30", "S3 Format 此站執行_31", "S3 Format OK_32", "S3 Format NG_33", "S3 燒入程式 此站執行_34", "S3 燒入程式 OK_35", "S3 燒入程式 NG_36", "S3 備用_37", "S3 備用_38", "S3 動作完成_39", "S4 PC動作中_40", "S4 量測完成 產品正常_41", "S4 量測完成 產品NG_42", "S4 Format 此站執行_43", "S4 Format OK_44", "S4 Format NG_45", "S4 燒入 此站不執行_46", "S4 燒入程式 OK_47", "S4 燒入程式 NG_48", "S4 藍芽Scan OK_49", "S4 藍芽Scan NG_50", "S4 動作完成_51", "給PLC要量電流訊號", "給PLC要量電壓訊號"]
                        n244 = call "Set OutputPLC.vi"("Array"=w508, "Address In"=20) -> ("Error Out"=w506:errorcluster[])  [unwired: 9 in]
                      }
                      frame True {
                        w510 = T8[] [enum."電流量測完成產品OK_21"] items=["S2站PC動作中_20", "電流量測完成產品OK_21", "電流量測完成產品NG_22", "S2站Format 執行_23", "S2 Format OK_24", "S2 Format NG_25", "S2站燒入執行_26", "S2站燒入OK_27", "S2站燒入NG_28", "S2站動作完成_29", "S3 PC動作中_30", "S3 Format 此站執行_31", "S3 Format OK_32", "S3 Format NG_33", "S3 燒入程式 此站執行_34", "S3 燒入程式 OK_35", "S3 燒入程式 NG_36", "S3 備用_37", "S3 備用_38", "S3 動作完成_39", "S4 PC動作中_40", "S4 量測完成 產品正常_41", "S4 量測完成 產品NG_42", "S4 Format 此站執行_43", "S4 Format OK_44", "S4 Format NG_45", "S4 燒入 此站不執行_46", "S4 燒入程式 OK_47", "S4 燒入程式 NG_48", "S4 藍芽Scan OK_49", "S4 藍芽Scan NG_50", "S4 動作完成_51", "給PLC要量電流訊號", "給PLC要量電壓訊號"]
                        n245 = call "Set OutputPLC.vi"("Array"=w510, "Address In"=20) -> ("Error Out"=w509:errorcluster[])  [unwired: 9 in]
                      }
                    }
                  }
                  frame Enabled {
                  }
                }
                n246 = call "Red PLC InReg.vi"("length"=10, "Input Registers Arr"=w480) -> ("Rad In Reg"=w479:string)  [unwired: 8 in, 1 out]
                n247 = call "Cub Meaasure FGV.vi"("Action"=Table_Save."Write" ("Enum"), 7:MeasureDisplayTab."耗電流 uA(電流表)", "DataIn"=w474, "SN"=w479) -> ()  [unwired: 5 in, 7 out]
                n248 = Merge Errors(w472, w471) -> (w470:errorcluster)
              }
              frame "T2" {
                w544 = u16 3 items=["SYSTem:VERSion?", "SYSTem:ERRor?", "*IDN?", "MEAS:CURR:DC?", "MEAS:VOLT?", "SYSTem:ERRor?"] ("Ringfor34450A")
                w543 = u16 5 items=["SYSTem:VERSion?", "SYSTem:ERRor?", "*IDN?", "MEAS:CURR:DC?", "MEAS:VOLT?", "MEAS:VOLT:DC?"] ("RingforIT8511")
                w541 = u16 0 items=["IT8511", "34450A", "WRBuff"] ("ChangeStatus")
                # "收尋S2站條碼"
                # "量電壓"
                n249 = call "Auto Inspection_Status.vi"("Action"=enum16{"Initial", "Write", "Read"}."Write", "DataIn"="IT8511", "Station"=Auto_Inspection_Station_Name2."S2Measure", "Data"=Auto_Inspection_Data_Name."CurrentAction") -> ()  [unwired: 9 in, 3 out]
                n250 = call "Retry Num.vi"("String"=w535) -> ("Numeric"=w549:i32, "retry次數"=w548:string[])  [unwired: 9 in]
                n251 = local write "retry次數"(w548) -> ()
                n252 = local write "Retry"(w549) -> ()
                n253 = call "MTool34450A.vi"("Ringfor34450A"=w544, "RingforIT8511"=w543, "VISA resource name"=refnum<visa-resource-name> "COM11", "ChangeStatus"=w541) -> ("error out"=w545:errorcluster, "μA"=→"T2 μA":dbl, "read buffer"=w522:string)  [unwired: 4 in, 1 out]
                "T2 buffer" <- w522
                n254 = Unbundle By Name(w545) -> ("status"=w516:bool)
                n255 = Increment(x=w536) -> (x+1=w518:i32)
                n256 = Not(x=w516) -> (.not. x?=w517:bool)
                n257 = Select(t=w518, s=w516, f=w518) -> (s? t:f=w547:i32)
                n258 = Greater Or Equal?(x=w547, y=w549) -> (x >= y?=w546:bool)
                n259 = Increment(x=w537) -> (x+1=w550:i32)
                n260 = Select(t=w522, s=w517, f="NG" ("DataIn")) -> (s? t:f=w523:string)
                n261 = global read "Main Glb.vi" "Input Registers0-99"() -> (w530:u16[])
                n262 = Select(t=w550, s=w517, f=w537) -> (s? t:f=w538:i32)
                n263 = case shown="False" w546 {
                  tunnel: [errorcluster {"status"=FALSE, "code"=0, "source"=""} ("error constant") w562] -> w520
                  tunnel: w547 -> [w560 _]
                  tunnel: [w560 0] -> w540
                  tunnel: w545 -> [_ w562]
                  frame False {
                  }
                  frame True {
                  }
                }
                n264 = disable-structure shown="Disabled" {
                  disable-tunnel: [w553 _] -> w521
                  disable-tunnel: w517 -> [w552 _]
                  frame Disabled {
                    n265 = case shown="True" w552 {
                      tunnel: [w554 w557] -> w553
                      frame False {
                        w556 = T8[] [enum."S4 量測完成 產品NG_42"] items=["S2站PC動作中_20", "電流量測完成產品OK_21", "電流量測完成產品NG_22", "S2站Format 執行_23", "S2 Format OK_24", "S2 Format NG_25", "S2站燒入執行_26", "S2站燒入OK_27", "S2站燒入NG_28", "S2站動作完成_29", "S3 PC動作中_30", "S3 Format 此站執行_31", "S3 Format OK_32", "S3 Format NG_33", "S3 燒入程式 此站執行_34", "S3 燒入程式 OK_35", "S3 燒入程式 NG_36", "S3 備用_37", "S3 備用_38", "S3 動作完成_39", "S4 PC動作中_40", "S4 量測完成 產品正常_41", "S4 量測完成 產品NG_42", "S4 Format 此站執行_43", "S4 Format OK_44", "S4 Format NG_45", "S4 燒入 此站不執行_46", "S4 燒入程式 OK_47", "S4 燒入程式 NG_48", "S4 藍芽Scan OK_49", "S4 藍芽Scan NG_50", "S4 動作完成_51", "給PLC要量電流訊號", "給PLC要量電壓訊號"]
                        n266 = call "Set OutputPLC.vi"("Array"=w556, "Address In"=20) -> ("Error Out"=w554:errorcluster[])  [unwired: 9 in]
                      }
                      frame True {
                        w558 = T8[] [enum."S4 量測完成 產品正常_41"] items=["S2站PC動作中_20", "電流量測完成產品OK_21", "電流量測完成產品NG_22", "S2站Format 執行_23", "S2 Format OK_24", "S2 Format NG_25", "S2站燒入執行_26", "S2站燒入OK_27", "S2站燒入NG_28", "S2站動作完成_29", "S3 PC動作中_30", "S3 Format 此站執行_31", "S3 Format OK_32", "S3 Format NG_33", "S3 燒入程式 此站執行_34", "S3 燒入程式 OK_35", "S3 燒入程式 NG_36", "S3 備用_37", "S3 備用_38", "S3 動作完成_39", "S4 PC動作中_40", "S4 量測完成 產品正常_41", "S4 量測完成 產品NG_42", "S4 Format 此站執行_43", "S4 Format OK_44", "S4 Format NG_45", "S4 燒入 此站不執行_46", "S4 燒入程式 OK_47", "S4 燒入程式 NG_48", "S4 藍芽Scan OK_49", "S4 藍芽Scan NG_50", "S4 動作完成_51", "給PLC要量電流訊號", "給PLC要量電壓訊號"]
                        n267 = call "Set OutputPLC.vi"("Array"=w558, "Address In"=20) -> ("Error Out"=w557:errorcluster[])  [unwired: 9 in]
                      }
                    }
                  }
                  frame Enabled {
                  }
                }
                n268 = call "Red PLC InReg.vi"("length"=10, "index"=10, "Input Registers Arr"=w530) -> ("Rad In Reg"=w529:string)  [unwired: 7 in, 1 out]
                n269 = call "Cub Meaasure FGV.vi"("Action"=Table_Save."Write" ("Enum"), 7:MeasureDisplayTab."電池負載電壓", "DataIn"=w523, "SN"=w529) -> ()  [unwired: 5 in, 7 out]
                n270 = Merge Errors(w521, w520) -> (w519:errorcluster)
              }
            }
          }
          frame True {
            w564 = TRUE
            "Boolean" <- w564
          }
        }
        n271 = property class="DigNum (strict)"(reference=w68, "Value"=w67) -> ()  [unwired: 1 in, 2 out]
        n272 = Compound Arithmetic op=OR(w65, w72, "stop") -> (w71:bool)
      }
    }
    frame Enabled {
    }
  }
  n273 = disable-structure shown="Disabled" {
    frame Disabled {
    }
    frame Enabled {
    }
  }
  n274 = disable-structure shown="Disabled" {
    frame Disabled {
      n275 = call "Save Table Test.vi"() -> ()  [unwired: 10 in, 2 out]
    }
    frame Enabled {
    }
  }
  n276 = disable-structure shown="Disabled" {
    frame Disabled {
      n277 = while {
        tunnel: cluster{"Table Control":string[][]}[] [{"Table Control"=[]}] ("Array 2") -> [w572]
        shift-right: [w571] -> w565
        shift-left: _ -> [w569]
        stop <- TRUE stop-if-true
        n278 = case shown="\"Add\"" "Enum" {
          tunnel: w572 -> [w574 _ _ _ _ _]
          tunnel: [w574 w578 w583 w608 w630 w637] -> w571
          tunnel: "Table Control 3" -> [_ w576 w585 w599 _ _]
          tunnel: w569 -> [_ w575 w580 w606 w629 w637]
          tunnel: "SN" -> [_ _ w579 w605 w628 _]
          frame "initial", Default {
          }
          frame "Add" {
            n279 = Bundle("Table Control 3"=w576) -> (w577:cluster{"Table Control 3":string[][]})  [unwired: 1 in]
            n280 = Build Array (concatenate)(w575, w577) -> (w578:cluster{"Table Control 3":string[][]}[])
            n281 = Bundle() -> ()  [unwired: 2 in, 1 out]
          }
          frame "Write" {
            n282 = for {
              tunnel: w580 -> [w593] mode=indexing
              tunnel: [w589] -> w588 mode=indexing
              n283 = Unbundle By Name(w593) -> ("Table Control 3"=w592:string[][])
              n284 = Index Array(array=w592, index (row)=0 ("disabled index (col)"), index (col)=1 ("disabled index (col)")) -> (element=w589:string)
            }
            n285 = Search 1D Array(1D array=w588, element=w579) -> (index of element=w584:i32)  [unwired: 1 in]
            n286 = Index Array(array=w580, index=w584) -> (element=w587:cluster{"Table Control 3":string[][]})
            n287 = Unbundle By Name(w587) -> ("Table Control 3"=w586:string[][])
            n288 = Build Array (concatenate)(w586, w585) -> (w582:string[][])
            n289 = Bundle(w582) -> (w581:cluster{string[][]})  [unwired: 1 in]
            n290 = Replace Array Subset(array=w580, new element=w581, index=w584) -> (w583:cluster{"Table Control 3":string[][]}[])
          }
          frame "Replace" {
            n291 = for {
              tunnel: w606 -> [w622] mode=indexing
              tunnel: [w618] -> w610 mode=indexing
              n292 = Unbundle By Name(w622) -> ("Table Control 3"=w621:string[][])
              n293 = Index Array(array=w621, index (row)=0 ("disabled index (col)"), index (col)=1 ("disabled index (col)")) -> (element=w618:string)
            }
            n294 = Search 1D Array(1D array=w610, element=w605) -> (index of element=w603:i32)  [unwired: 1 in]
            n295 = Index Array(array=w606, index=w603) -> (element=w609:cluster{"Table Control 3":string[][]})
            n296 = Unbundle By Name(w609) -> ("Table Control 3"=w596:string[][])
            n297 = Array Size(array=w599) -> (size(s)=w601:i32[])
            n298 = Index Array(array=w599, index (col)=1 ("disabled index (col)")) -> (element=w597:string[])  [unwired: 1 in]
            n299 = Index Array(array=w601) -> (element #1=w600:i32)  [unwired: 2 in, 1 out]
            n300 = Array Size(array=w596) -> (size(s)=w602:i32[])
            n301 = Index Array(array=w602) -> (element #1=w595:i32)  [unwired: 2 in, 1 out]
            n302 = Subtract(x=w595, y=w600) -> (x-y=w594:i32)
            n303 = for {
              shift-right: [w617] -> w604
              shift-left: w596 -> [w616]
              tunnel: w594 -> [w613]
              tunnel: w597 -> [w612] mode=indexing
              i -> [w614]
              n304 = Add(x=w613, y=w614) -> (x+y=w611:i32)
              n305 = Replace Array Subset(array=w616, new element=w612, index (row)=w611, index (col)=1 ("disabled index (col)")) -> (w617:string[][])
            }
            n306 = Bundle("Table Control 3"=w604) -> (w607:cluster{"Table Control 3":string[][]})  [unwired: 1 in]
            n307 = Replace Array Subset(array=w606, new element=w607, index=w603) -> (w608:cluster{"Table Control 3":string[][]}[])
          }
          frame "Delete" {
            n308 = for {
              tunnel: w629 -> [w636] mode=indexing
              tunnel: [w632] -> w631 mode=indexing
              n309 = Unbundle By Name(w636) -> ("Table Control 3"=w635:string[][])
              n310 = Index Array(array=w635, index (row)=0 ("disabled index (col)"), index (col)=1 ("disabled index (col)")) -> (element=w632:string)
            }
            n311 = Search 1D Array(1D array=w631, element=w628) -> (index of element=w627:i32)  [unwired: 1 in]
            n312 = Index Array(array=w629, index=w627) -> ()  [unwired: 1 out]
            n313 = Delete From Array(array=w629, length=1, index=w627) -> (deleted portion=w625:cluster{"Table Control 3":string[][]}[], array with subset deleted=w630:cluster{"Table Control 3":string[][]}[])
            n314 = Index Array(array=w625) -> (element=w624:cluster{"Table Control 3":string[][]})  [unwired: 1 in]
            n315 = Unbundle By Name(w624) -> ("Table Control 3"=→"LOG":string[][])
          }
          frame "REad" {
          }
        }
      }
      "Array 3" <- w565
    }
    frame Enabled {
    }
  }
